vi "strcpy.vi"(4 "error in (no error)":errorcluster, 6 "lpString2 (NULL)\n[SOURCE]":i32 format="%.0x", 7 "lpString1 (NULL)\n[TARGET]":i32 format="%.0x") -> (0 "error out":errorcluster, 3 "lpString1":i32 format="%.0x")   [LabVIEW 2011]
uses:
  KERNEL32.DLL
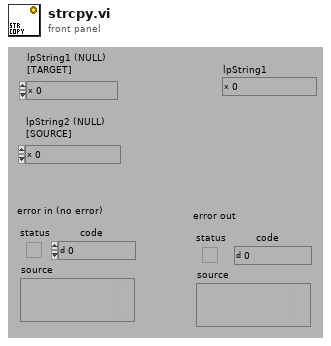
[diagram p1: front panel]
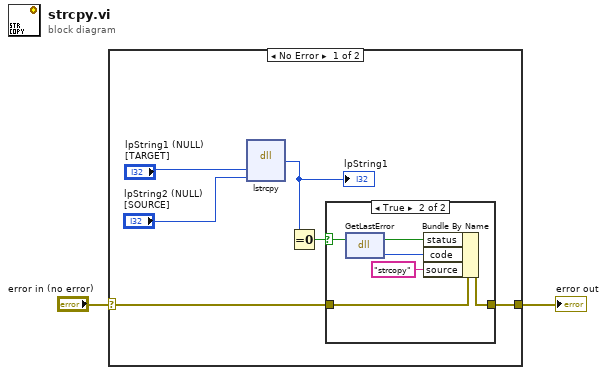
[diagram p0: block diagram]
diagram:
  n1 = case shown="No Error" "error in (no error)" {
    selector: "error in (no error)" -> [w7 w15]
    tunnel: [w6 w15] -> w1
    frame No Error {
      n2 = dll-call lib="KERNEL32.DLL" fn="lstrcpy" label="LPTSTR lstrcpy(\n  LPTSTR lpString1,  // pointer to buffer\n  LPCTSTR lpString2  // pointer to string to copy\n);"("lpString1"="lpString1 (NULL)\n[TARGET]", "lpString2"="lpString2 (NULL)\n[SOURCE]") -> ("LPSTR"=w5:i32)  [unwired: 5 in, 2 out]
      "lpString1" <- w5
      n3 = Equal To 0?(x=w5) -> (x = 0?=w8:bool)
      n4 = case shown="True" w8 {
        selector: w8 -> [_ w13]
        tunnel: w7 -> [w9 w14]
        tunnel: [w9 w12] -> w6
        frame False {
        }
        frame True {
          n5 = dll-call lib="KERNEL32.DLL" fn="GetLastError"() -> (w10:i32)  [unwired: 3 in, 2 out]
          n6 = Bundle By Name(cluster=w14, "status"=w13, "code"=w10, "source"="strcopy") -> (w12:errorcluster)
        }
      }
    }
    frame Error {
    }
  }
  "error out" <- w1
